vi "Generate_trial_sequence.vi"(9 "Repeats":u32, 10 "Protocol cluster":T1, 11 "Sequences":T2(array[cluster])) -> (3 "Array":cluster{"Sequence name":string, "Active":bool}[](array[cluster]))   [LabVIEW 2016]
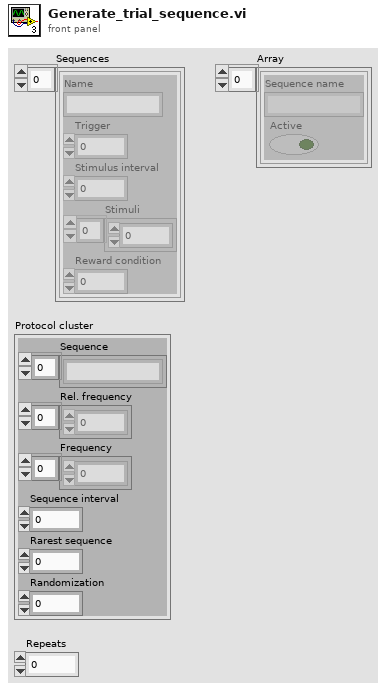
[diagram p1: front panel]
types:
  T1 = cluster{"Sequence":string[], "Rel. frequency":u32[], "Frequency":dbl[], "Sequence interval":dbl, "Rarest sequence ":dbl, "Randomization":u16}
  T2 = cluster{"Name":string, "Trigger":u16, "Stimulus interval":dbl, "Stimuli":i32[], "Reward condition":u16}[]
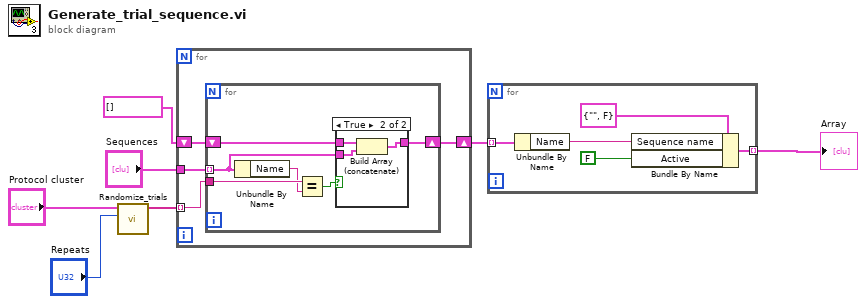
[diagram p0: block diagram]
diagram:
  n1 = call "Randomize_trials.vi"("Repeats"="Repeats", "Protocol cluster"="Protocol cluster") -> ("Trials"=w3:string[])  [unwired: 9 in]
  n2 = for {
    tunnel: w3 -> [w10] mode=indexing
    tunnel: "Sequences" -> [w11]
    shift-right: [w8] -> w6
    shift-left: T2 [] -> [w9]
    n3 = for {
      tunnel: w11 -> [w15] mode=indexing
      tunnel: w10 -> [w17]
      shift-right: [w13] -> w8
      shift-left: w9 -> [w14]
      n4 = Unbundle By Name(w15) -> ("Name"=w16:string)
      n5 = Equal?(x=w17, y=w16) -> (x = y?=w12:bool)
      n6 = case shown="True" w12 {
        tunnel: w15 -> [_ w20]
        tunnel: w14 -> [w18 w21]
        tunnel: [w18 w19] -> w13
        frame False {
        }
        frame True {
          n7 = Build Array (concatenate)(w21, w20) -> (w19:T2)
        }
      }
    }
  }
  n8 = for {
    tunnel: w6 -> [w26] mode=indexing
    tunnel: [w22] -> w7 mode=indexing
    n9 = Unbundle By Name(w26) -> ("Name"=w24:string)
    n10 = Bundle By Name(cluster=cluster{"Sequence name":string, "Active":bool} {"Sequence name"="", "Active"=FALSE} ("Cluster"), "Sequence name"=w24, "Active"=FALSE) -> (w22:cluster{"Sequence name":string, "Active":bool})
  }
  "Array" <- w7
